vi "rate_limit.vi"(10 "Max Delta Per Iteration":dbl, 11 "Drive":cluster{"Left":dbl, "Right":dbl}) -> (3 "Output":cluster{"Left":dbl, "Right":dbl})   [LabVIEW 2011]
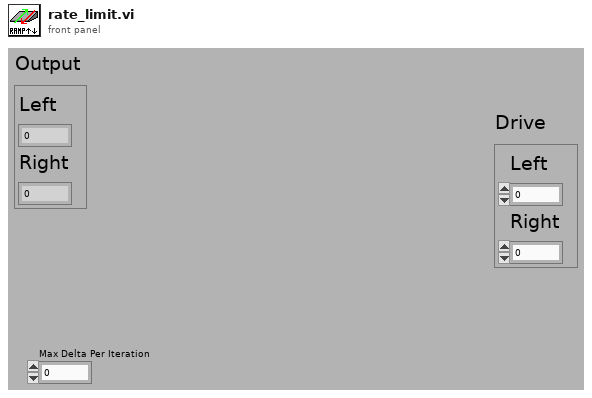
[diagram p1: front panel]
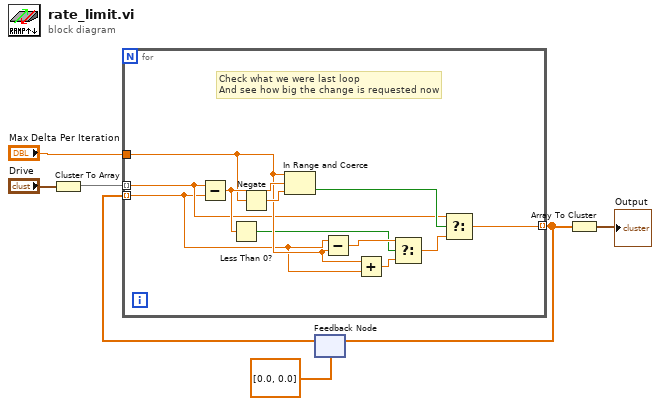
[diagram p0: block diagram]
diagram:
  n1 = Cluster To Array(cluster="Drive") -> (array=w5:dbl[])
  n2 = feedback #1(dbl[] [0.0, 0.0]) -> (w4:dbl[])
  n3 = for {
    tunnel: w5 -> [w10] mode=indexing
    tunnel: w4 -> [w8] mode=indexing
    tunnel: "Max Delta Per Iteration" -> [w11]
    tunnel: [w16] -> w2 mode=indexing
    # "Check what we were last loop\nAnd see how big the change is requested now"
    n4 = Subtract(x=w10, y=w8) -> (x-y=w14:dbl)
    n5 = Less Than 0?(x=w14) -> (x < 0?=w9:bool)
    n6 = Negate(x=w11) -> (-x=w18:dbl)
    n7 = In Range and Coerce(upper limit=w11, x=w14, lower limit=w18) -> (In Range?=w17:bool)  [unwired: 1 out]
    n8 = Subtract(x=w8, y=w11) -> (x-y=w13:dbl)
    n9 = Add(x=w11, y=w8) -> (x+y=w12:dbl)
    n10 = Select(t=w13, s=w9, f=w12) -> (s? t:f=w15:dbl)
    n11 = Select(t=w10, s=w17, f=w15) -> (s? t:f=w16:dbl)
  }
  n12 = feedback-in #1(w2) -> ()
  n13 = Array To Cluster(array=w2) -> (cluster=→"Output":cluster{"[0]":dbl, "[1]":dbl})
